vi "Wait For DAQ to Start.vi"(8 "error in (no error)":errorcluster) -> (0 "error out":errorcluster)   [LabVIEW 2020]
uses:
  PXI Globals.vi
panel:
  in  "Refresh (ms)":dbl=5.0
  in  "Timeout (ms)":dbl=5000.0
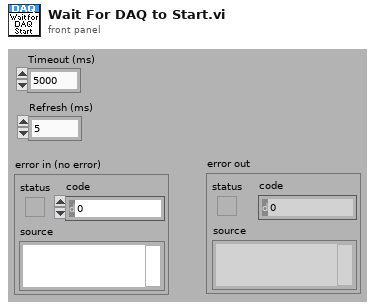
[diagram p1: front panel]
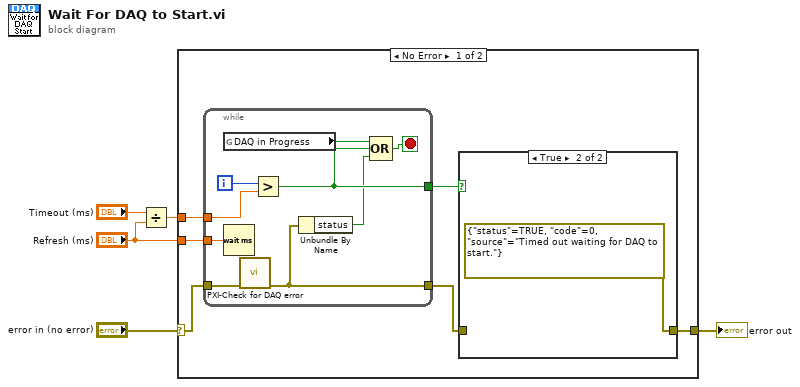
[diagram p0: block diagram]
diagram:
  n1 = Divide(x="Timeout (ms)", y="Refresh (ms)") -> (x/y=w1:dbl)
  n2 = case shown="No Error" "error in (no error)" {
    selector: "error in (no error)" -> [w7 w23]
    tunnel: [w8 w23] -> w4
    tunnel: "Refresh (ms)" -> [w11 _]
    tunnel: w1 -> [w10 _]
    frame No Error {
      n3 = while {
        tunnel: w11 -> [w22]
        tunnel: w10 -> [w20]
        tunnel: [w17] -> w9
        tunnel: w7 -> [w16]
        tunnel: [w14] -> w6
        i -> [w21]
        stop <- w18 stop-if-true
        n4 = global read "PXI Globals.vi" "DAQ in Progress"() -> (w19:bool)
        n5 = Wait (ms)(milliseconds to wait=w22) -> ()  [unwired: 1 out]
        n6 = call "PXI-Check for DAQ error.vi"("error in (no error)"=w16) -> ("error out"=w14:errorcluster)  [unwired: 14 in]
        n7 = Greater?(x=w21, y=w20) -> (0:w17:bool)
        n8 = Unbundle By Name(w14) -> ("status"=w15:bool)
        n9 = Compound Arithmetic op=OR(w19, w17, w15) -> (w18:bool)
      }
      n10 = case shown="True" w9 {
        tunnel: w6 -> [w12 _]
        tunnel: [w12 errorcluster {"status"=TRUE, "code"=0, "source"="Timed out waiting for DAQ to start."} ("error IO")] -> w8
        frame False {
        }
        frame True {
        }
      }
    }
    frame Error {
    }
  }
  "error out" <- w4
